vi "Two_sine_waves_of_variable__phase.vi"() -> ()   [LabVIEW 2020]
uses:
  <vilib>/Analysis/NI_AALPro.lvlib
panel:
  out "phase":i32
  out "R":dbl format="%0.2f"
  out "DC Sine (X)":dbl format="%0.2f"
  out "DC Sine (Y)":dbl format="%0.2f"
  in  "?":bool
  out "Input Phase difference":i32
  out "Waveform Chart 2":cluster{dbl, dbl}(graph)
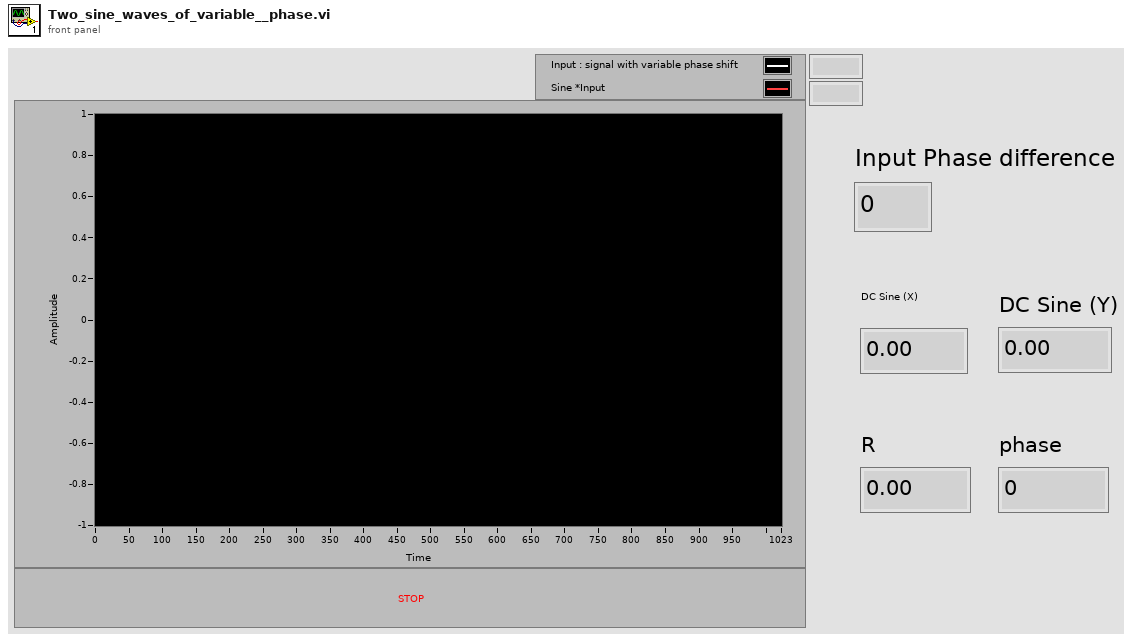
[diagram p1: front panel]
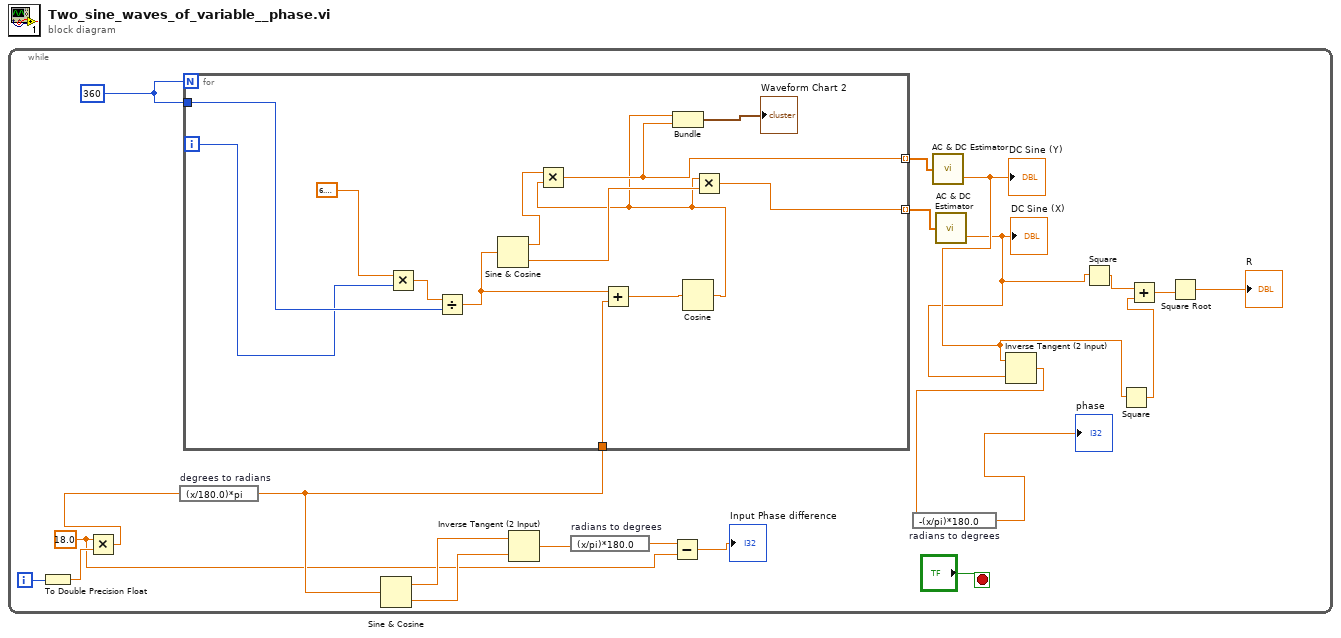
[diagram p0: block diagram]
diagram:
  n1 = while {
    i -> [w19]
    stop <- "?" stop-if-true
    w1 = 18.0 ("x")
    w22 = 360
    n2 = To Double Precision Float(number=w19) -> (double precision float=w18:dbl)
    n3 = Multiply(x=w1, y=w18) -> (x*y=w20:dbl)
    n4 = expression code="(x/180.0)*pi" "degrees to radians"(w20) -> (w11:dbl)
    n5 = for {
      N: w22 -> [_]
      tunnel: w22 -> [w33]
      tunnel: [w27] -> w17 mode=indexing
      tunnel: [w26] -> w16 mode=indexing
      tunnel: w11 -> [w23]
      i -> [w32]
      n6 = Multiply(x=6.283185307179586, y=w32) -> (x*y=w35:dbl)
      n7 = Divide(x=w35, y=w33) -> (x/y=w30:dbl)
      n8 = Sine & Cosine(0:w30) -> (1:w29:dbl, 2:w28:dbl)
      n9 = Add(x=w30, y=w23) -> (x+y=w25:dbl)
      n10 = Cosine(x=w25) -> (cos(x)=w24:dbl)
      n11 = Multiply(x=w29, y=w24) -> (x*y=w27:dbl)
      n12 = Bundle(w24, w27) -> (→"Waveform Chart 2":cluster{dbl, dbl})  [unwired: 1 in]
      n13 = Multiply(x=w24, y=w28) -> (x*y=w26:dbl)
    }
    n14 = Sine & Cosine(0:w11) -> (1:w12:dbl, 2:w13:dbl)
    n15 = Inverse Tangent (2 Input)(1:w13, 2:w12) -> (0:w10:dbl)
    n16 = expression code="(x/pi)*180.0" "radians to degrees"(w10) -> (w3:dbl)
    n17 = Subtract(x=w3, y=w1) -> (x-y=→"Input Phase difference":dbl)
    n18 = call <vilib>:"AC & DC Estimator.vi"("Signal (V)"=w17) -> ("DC estimate (V)"=w9:dbl)  [unwired: 1 out]
    "DC Sine (Y)" <- w9
    n19 = call <vilib>:"AC & DC Estimator.vi"("Signal (V)"=w16) -> ("DC estimate (V)"=w8:dbl)  [unwired: 1 out]
    "DC Sine (X)" <- w8
    n20 = Inverse Tangent (2 Input)(1:w8, 2:w9) -> (0:w14:dbl)
    n21 = expression code="-(x/pi)*180.0" "radians to degrees"(w14) -> (→"phase":dbl)
    n22 = Square(x=w8) -> (x^2=w6:dbl)
    n23 = Square(x=w9) -> (x^2=w7:dbl)
    n24 = Add(x=w6, y=w7) -> (x+y=w5:dbl)
    n25 = Square Root(x=w5) -> (sqrt(x)=→"R":dbl)
  }
